vi "UpdateMotors_BulldozerDrive.vi"(1 "Max Duty Cycle":dbl min=-1.0 max=1.0 step=0.001, 2 "RMot":dbl min=-1.0 max=1.0 step=0.01, 3 "LMot":dbl min=-1.0 max=1.0 step=0.001, 4 "PWM Offset":dbl=0.4 format="%#_13g", 5 "Motor PWMs":T8) -> ()   [LabVIEW 2015]
uses:
  <vilib>/myRIO/Instrument Drivers/Onboard IO/PWM/typedefs/PWM Reference.ctl
  <vilib>/myRIO/Common/Instrument Driver Framework/Utilities/typedefs/myRIO Generic Hardware Reference.ctl
  <vilib>/myRIO/Common/Instrument Driver Framework/Utilities/typedefs/Hardware Version Enum.ctl
  <vilib>/myRIO/Common/Instrument Driver Framework/Utilities/typedefs/myRIO v1.0 Reference.ctl
  <vilib>/myRIO/Common/Instrument Driver Framework/Utilities/typedefs/Generic FPGA Reference.ctl
  <vilib>/myRIO/Common/Instrument Driver Framework/myRIO v1.0/PWM/typedefs/PWM Channels Enum.ctl
  <vilib>/myRIO/Instrument Drivers/Onboard IO/PWM/typedefs/PWM Configuration.ctl
  <vilib>/myRIO/Instrument Drivers/Onboard IO/PWM/PWM.lvlib
panel:
  out "LMotF":dbl(graph)
  # "UpdateMotors_BulldozerDrive"
  # "The UpdateMotors_BulldozerDrive.vi is a modification of the \nupdate motors vi from the fall semester of ant robot research.\n\nThe big change is that this VI takes in 1 value for each motor.\nThis value is between [-1,1], where -1 drives that wheel fullspeed backwards,\nand 1] drives that motor full speed foward.  \n\nThe Duty cycle value to each motor is offset by PWM offset towards making that \nwheel move in its desired direction.\n\n\nNOTE: Charts can be removed to optimize code."
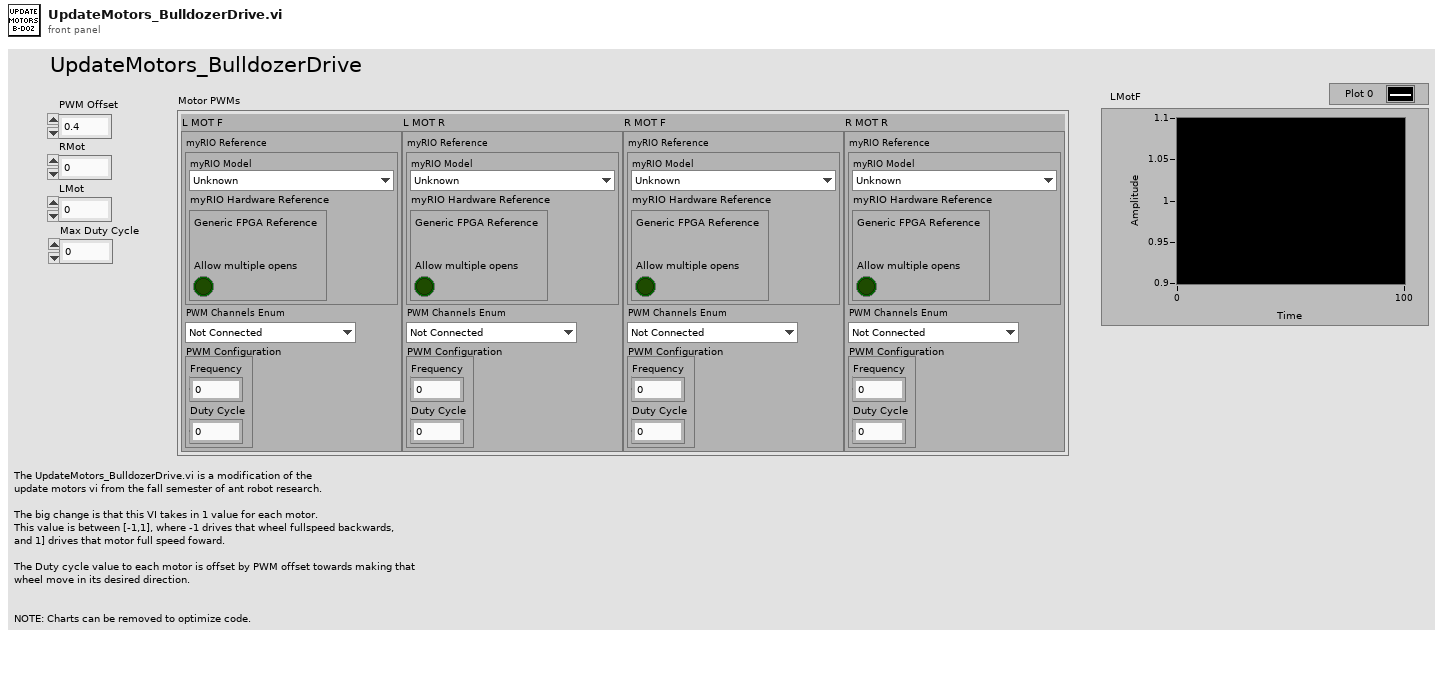
[diagram p1: front panel]
types:
  T1 = typedef "PWM.lvlib/PWM Reference.ctl" = cluster{"myRIO Reference":T2, "PWM Channels Enum":T6, "PWM Configuration":T7}
  T2 = typedef "myRIO Generic Hardware Reference.ctl" = cluster{"myRIO Model":T3, "myRIO Hardware Reference":T4}
  T3 = typedef "Hardware Version Enum.ctl" = enum16{"Unknown", "myRIO-1900", "myRIO-1950", "roboRIO"}
  T4 = typedef "myRIO v1.0 Reference.ctl" = cluster{"Generic FPGA Reference":T5, "Allow multiple opens":bool}
  T5 = typedef "Generic FPGA Reference.ctl" = refnum<k20>
  T6 = typedef "PWM Channels Enum.ctl" = enum16{"Not Connected", "C/PWM0", "C/PWM1", "A/PWM0", "A/PWM1", "A/PWM2", "B/PWM0", "B/PWM1", "B/PWM2", "PWM/PWM0", "PWM/PWM1", "PWM/PWM2", "PWM/PWM3", "PWM/PWM4", "PWM/PWM5", "PWM/PWM6", "PWM/PWM7", "PWM/PWM8", "PWM/PWM9"}
  T7 = typedef "PWM.lvlib/PWM Configuration.ctl" = cluster{"Frequency":dbl, "Duty Cycle":dbl}
  T8 = cluster{"L MOT F ":T1, "L MOT R":T1, "R MOT F":T1, "R MOT R":T1}
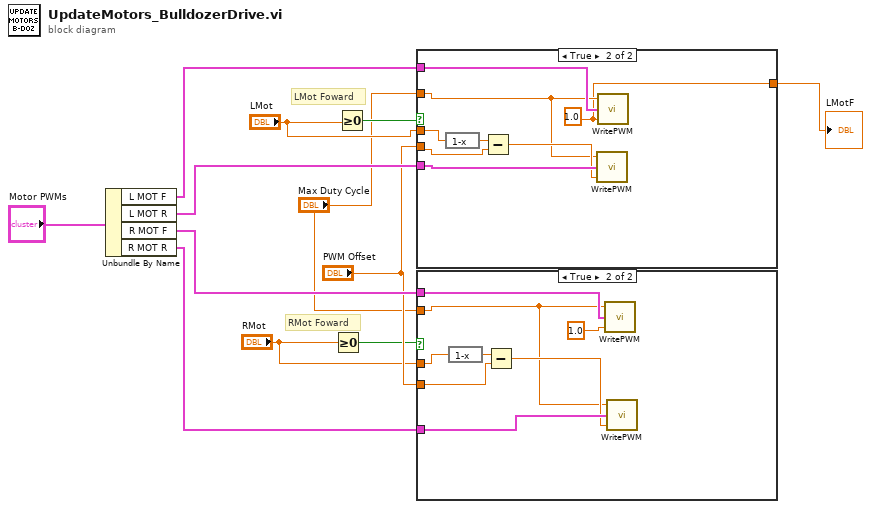
[diagram p0: block diagram]
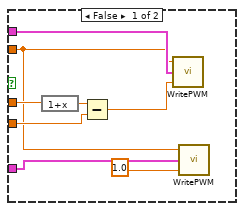
[diagram p2: hidden frame]
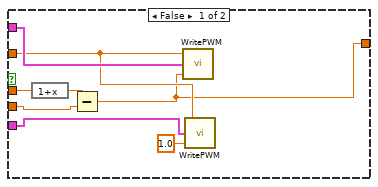
[diagram p3: hidden frame]
diagram:
  # "LMot Foward"
  # "RMot Foward"
  n1 = Unbundle By Name("Motor PWMs") -> ("L MOT F"=w11:T1, "L MOT R"=w10:T1, "R MOT F"=w9:T1, "R MOT R"=w8:T1)
  n2 = Greater Or Equal To 0?(x="RMot") -> (x >= 0?=w6:bool)
  n3 = Greater Or Equal To 0?(x="LMot") -> (x >= 0?=w4:bool)
  n4 = case shown="True" w4 {
    tunnel: w11 -> [w19 w27]
    tunnel: w10 -> [w20 w28]
    tunnel: "LMot" -> [w16 w26]
    tunnel: "PWM Offset" -> [w17 w24]
    tunnel: "Max Duty Cycle" -> [w14 w22]
    tunnel: [w13 w21] -> w1
    frame False {
      n5 = expression code="1+x"(w16) -> (w18:dbl)
      n6 = Subtract(x=w18, y=w17) -> (x-y=w13:dbl)
      n7 = call "WritePWM.vi"("Input Duty Cycle"=w13, "L MOT F"=w19, "Max Duty Cycle"=w14) -> ()  [unwired: 2 in]
      n8 = call "WritePWM.vi"("Input Duty Cycle"=1.0, "L MOT F"=w20, "Max Duty Cycle"=w14) -> ()  [unwired: 2 in]
    }
    frame True {
      w21 = 1.0
      n9 = expression code="1-x"(w26) -> (w25:dbl)
      n10 = Subtract(x=w25, y=w24) -> (x-y=w23:dbl)
      n11 = call "WritePWM.vi"("Input Duty Cycle"=w23, "L MOT F"=w28, "Max Duty Cycle"=w22) -> ()  [unwired: 2 in]
      n12 = call "WritePWM.vi"("Input Duty Cycle"=w21, "L MOT F"=w27, "Max Duty Cycle"=w22) -> ()  [unwired: 2 in]
    }
  }
  "LMotF" <- w1
  n13 = case shown="True" w6 {
    tunnel: w9 -> [w36 w43]
    tunnel: w8 -> [w35 w44]
    tunnel: "RMot" -> [w33 w40]
    tunnel: "PWM Offset" -> [w32 w39]
    tunnel: "Max Duty Cycle" -> [w29 w37]
    frame False {
      n14 = expression code="1+x"(w33) -> (w34:dbl)
      n15 = Subtract(x=w34, y=w32) -> (x-y=w30:dbl)
      n16 = call "WritePWM.vi"("Input Duty Cycle"=w30, "L MOT F"=w36, "Max Duty Cycle"=w29) -> ()  [unwired: 2 in]
      n17 = call "WritePWM.vi"("Input Duty Cycle"=1.0, "L MOT F"=w35, "Max Duty Cycle"=w29) -> ()  [unwired: 2 in]
    }
    frame True {
      n18 = expression code="1-x"(w40) -> (w42:dbl)
      n19 = Subtract(x=w42, y=w39) -> (x-y=w38:dbl)
      n20 = call "WritePWM.vi"("Input Duty Cycle"=1.0, "L MOT F"=w43, "Max Duty Cycle"=w37) -> ()  [unwired: 2 in]
      n21 = call "WritePWM.vi"("Input Duty Cycle"=w38, "L MOT F"=w44, "Max Duty Cycle"=w37) -> ()  [unwired: 2 in]
    }
  }
